vi "Read Coils from Slave.vi"(7 "Unit ID":u8, 8 "error in (no error)":errorcluster, 9 "length":u16, 10 "start":u16, 11 "Modbus Master in":refnum<class "Modbus Master.lvclass">) -> (0 "error out":errorcluster, 3 "coils":bool[](array[boolean]))   [LabVIEW 2020, in "Modbus Master Engine.lvlib"]
uses:
  Modbus Master Engine.lvlib
  Includes/Modbus API.lvlibp/API/Master/Modbus Master.lvclass
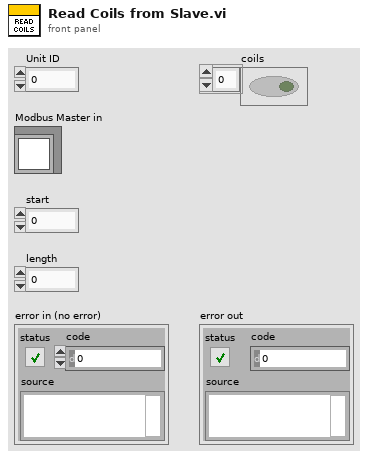
[diagram p1: front panel]
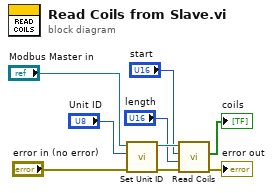
[diagram p0: block diagram]
diagram:
  n1 = call "Set Unit ID.vi"("error in"="error in (no error)", "unit ID"="Unit ID", "Modbus master in"="Modbus Master in") -> ("error out"=w7:errorcluster, "Modbus master out"=w6:refnum<class "Modbus Master.lvclass">)  [unwired: 7 in]
  n2 = call-dynamic "Read Coils.vi"("error in"=w7, "number of inputs"="length", "starting address"="start", "Modbus master in"=w6) -> ("error out"=→"error out":errorcluster, "coils"=→"coils":bool[])  [unwired: 5 in, 1 out]
